vi "xcorr_packet_U64 bkp.vi"(0 "x":u32, 1 "y":u32, 2 "trigger":bool) -> (8 "out":u64, 9 "valid":bool)   [LabVIEW 2017]
uses:
  <vilib>/rvi/FXPMathLib/basic elements/FxpDiscreteDelay/XNode/nifxpmath_DiscreteDelay.xnode
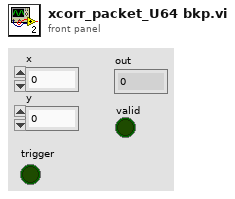
[diagram p1: front panel]
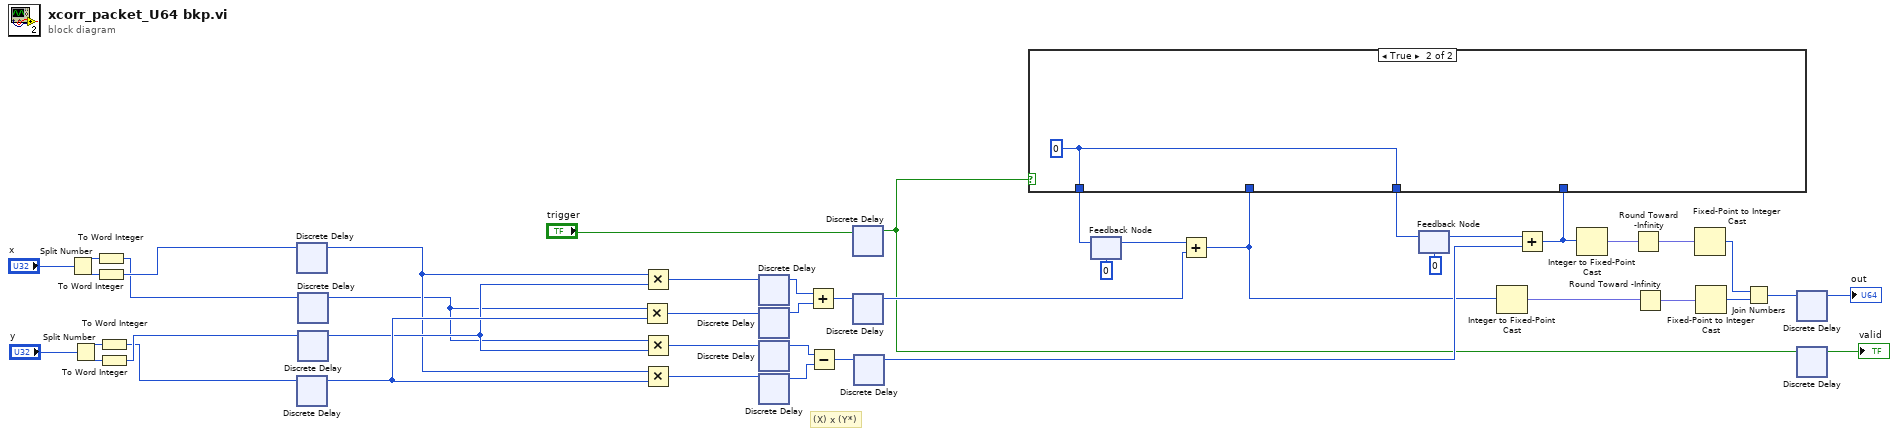
[diagram p0: block diagram]
diagram:
  # "(X) x (Y*)"
  n1 = Split Number(x="x") -> (hi(x)=w38:u16, lo(x)=w39:u16)
  n2 = Split Number(x="y") -> (hi(x)=w40:u16, lo(x)=w41:u16)
  n3 = To Word Integer(number=w38) -> (16bit integer=w21:i16)
  n4 = To Word Integer(number=w39) -> (16bit integer=w22:i16)
  n5 = To Word Integer(number=w40) -> (16bit integer=w19:i16)
  n6 = To Word Integer(number=w41) -> (16bit integer=w20:i16)
  n7 = xnode "Discrete Delay"("D"=w22) -> ("Q"=w26:i16)
  n8 = xnode "Discrete Delay"("D"=w19) -> ("Q"=w31:i16)
  n9 = xnode "Discrete Delay"("D"=w21) -> ("Q"=w25:i16)
  n10 = xnode "Discrete Delay"("D"=w20) -> ("Q"=w30:i16)
  n11 = Multiply(x=w25, y=w31) -> (x*y=w15:i32)
  n12 = Multiply(x=w26, y=w30) -> (x*y=w16:i32)
  n13 = Multiply(x=w25, y=w30) -> (x*y=w14:i32)
  n14 = Multiply(x=w26, y=w31) -> (x*y=w13:i32)
  n15 = xnode "Discrete Delay"("D"=w16) -> ("Q"=w32:i32)
  n16 = xnode "Discrete Delay"("D"=w15) -> ("Q"=w33:i32)
  n17 = xnode "Discrete Delay"("D"=w14) -> ("Q"=w34:i32)
  n18 = xnode "Discrete Delay"("D"=w13) -> ("Q"=w35:i32)
  n19 = Add(x=w32, y=w33) -> (x+y=w37:i32)
  n20 = Subtract(x=w34, y=w35) -> (x-y=w36:i32)
  n21 = xnode "Discrete Delay"("D"="trigger") -> ("Q"=w5:bool)
  n22 = xnode "Discrete Delay"("D"=w37) -> ("Q"=w18:i32)
  n23 = xnode "Discrete Delay"("D"=w36) -> ("Q"=w17:i32)
  n24 = feedback #1(i64 0) -> (w24:i64)
  n25 = Add(x=w24, y=w18) -> (x+y=w12:i64)
  n26 = feedback #2(i64 0) -> (w23:i64)
  n27 = Integer to Fixed-Point Cast(integer=w12) -> (fixed-point=w2:fxp<+/-,40,32>)  [unwired: 1 in]
  n28 = Add(x=w23, y=w17) -> (x+y=w10:i64)
  n29 = case shown="True" w5 {
    tunnel: [w47 w48] -> w28
    tunnel: [w46 w48] -> w27
    tunnel: w12 -> [w46 _]
    tunnel: w10 -> [w47 _]
    frame False {
    }
    frame True {
      w48 = i64 0
    }
  }
  n30 = feedback-in #1(w27) -> ()
  n31 = feedback-in #2(w28) -> ()
  n32 = Integer to Fixed-Point Cast(integer=w10) -> (fixed-point=w4:fxp<+/-,40,32>)  [unwired: 1 in]
  n33 = Round Toward -Infinity(1:w4) -> (0:w3:fxp<+/-,32,32>)
  n34 = Round Toward -Infinity(1:w2) -> (0:w1:fxp<+/-,32,32>)
  n35 = Fixed-Point to Integer Cast(1:w3) -> (0:w9:i32)
  n36 = Fixed-Point to Integer Cast(1:w1) -> (0:w11:i32)
  n37 = Join Numbers(hi=w9, lo=w11) -> ((hi.lo)=w8:u64)
  n38 = xnode "Discrete Delay"("D"=w8) -> ("Q"=→"out":u64)
  n39 = xnode "Discrete Delay"("D"=w5) -> ("Q"=→"valid":bool)
